vi "waitForReady.vi"(2 "axis":i32, 3 "errorIn":errorcluster, 4 "referenceIn":refnum<k24>) -> (0 "errorOut":errorcluster, 1 "referenceOut":refnum<k24>)   [LabVIEW 2020]
uses:
  C:/Program Files/Newport/Piezo Motion Control/Newport AG-UC2-UC8 Applet/Samples/LabVIEW 2009/AgilisCmdLib.dll
  Program Files/Newport/Piezo Motion Control/Newport AG-UC2-UC8 Applet/Samples/LabVIEW 2009/AgilisCmdLib.dll
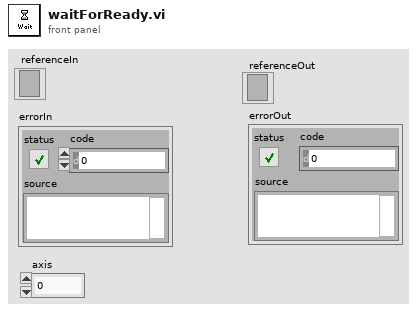
[diagram p1: front panel]
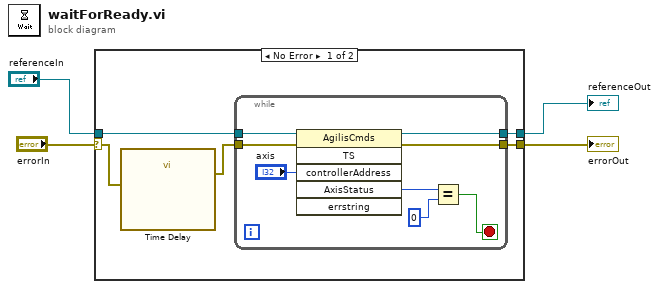
[diagram p0: block diagram]
diagram:
  n1 = case shown="No Error" "errorIn" {
    selector: "errorIn" -> [w6 w18]
    tunnel: [w9 w19] -> w4
    tunnel: [w8 w18] -> w3
    tunnel: "referenceIn" -> [w7 w19]
    frame No Error {
      n2 = call "Time Delay"("error in (no error)"=w6) -> ("error out"=w5:errorcluster)  [unwired: 10 in]
      n3 = while {
        tunnel: w7 -> [w17]
        tunnel: [w16] -> w9
        tunnel: [w15] -> w8
        tunnel: w5 -> [w13]
        stop <- w10 stop-if-true
        n4 = invoke class="AgilisCmds" method="TS"(reference=w17, error in=w13, "controllerAddress"="axis") -> (reference out=w16:refnum<k24>, error out=w15:errorcluster, "AxisStatus"=w12:i32)  [unwired: 3 in, 3 out]
        n5 = Equal?(x=w12, y=0) -> (x = y?=w10:bool)
      }
    }
    frame Error {
    }
  }
  "referenceOut" <- w4
  "errorOut" <- w3
